vi "MICSD Set Attenuator.vi"(8 "error in (no error)":errorcluster, 10 "Attenuation":u8, 11 "VISA Resource Name":refnum<visa-resource-name>) -> (0 "error out":errorcluster, 3 "dup VISA Resource Name":refnum<visa-resource-name>)   [LabVIEW 2020]
uses:
  <vilib>/Instr/_visa.llb/VISA Configure Serial Port (Instr).vi
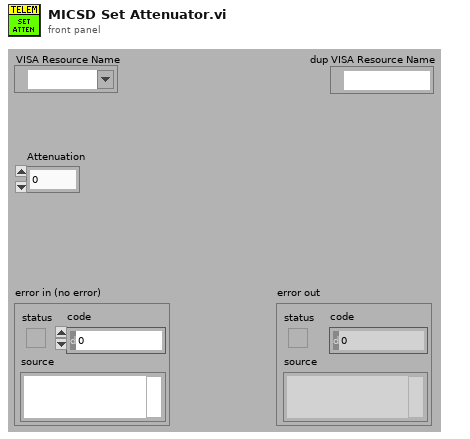
[diagram p1: front panel]
types:
  T1 = cluster{"Command Token":u8, "Length":u16, "Pack Data":u8[]}
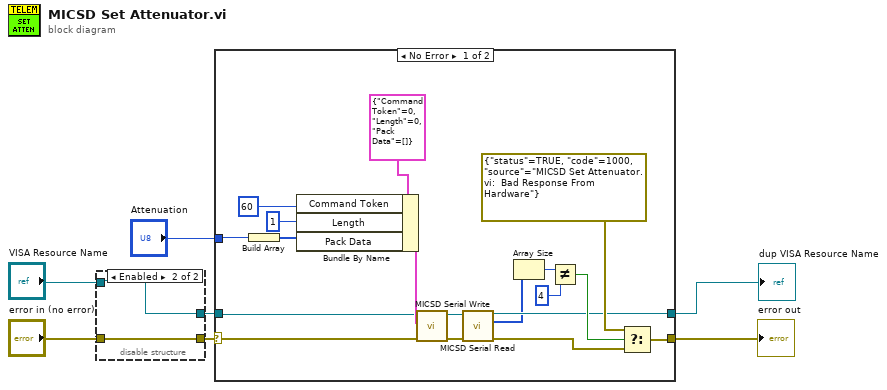
[diagram p0: block diagram]
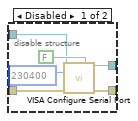
[diagram p2: hidden frame]
diagram:
  n1 = disable-structure shown="Enabled" {
    disable-tunnel: [w11 w14] -> w6
    disable-tunnel: "error in (no error)" -> [w10 w14]
    disable-tunnel: "VISA Resource Name" -> [w9 w15]
    disable-tunnel: [w8 w15] -> w3
    frame Disabled {
      n2 = call-poly "VISA Configure Serial Port"("VISA resource name"=w9, "Enable Termination\nChar (T)"=FALSE ("Enable Termination\nChar (T)"), "baud rate (9600)"=u32 230400, "error in (no error)"=w10) -> ("VISA resource name out"=w8:refnum<visa-resource-name>, "error out"=w11:errorcluster)  [unwired: 10 in]
    }
    frame Enabled {
    }
  }
  n3 = case shown="No Error" w6 {
    selector: w6 -> [w31 w35]
    tunnel: [w18 w35] -> w1
    tunnel: w3 -> [w30 w34]
    tunnel: [w21 w34] -> w7
    tunnel: "Attenuation" -> [w16 _]
    frame No Error {
      n4 = Build Array(w16) -> (w17:u8[])
      n5 = Bundle By Name(cluster=T1 {"Command Token"=0, "Length"=0, "Pack Data"=[]} ("Write Data"), "Command Token"=u16 60 ("Length"), "Length"=u16 1, "Pack Data"=w17) -> (w33:T1)
      n6 = call "MICSD Serial Write.vi"("error in (no error)"=w31, "Write Data"=w33, "VISA Resource Name"=w30) -> ("error out"=w27:errorcluster, "DUP Visa Resource Name"=w28:refnum<visa-resource-name>)  [unwired: 7 in]
      n7 = call "MICSD Serial Read.vi"("error in (no error)"=w27, "VISA Resource Name"=w28) -> ("error out"=w19:errorcluster, "Read Data"=w20:u8[], "DUP Visa Resource Name"=w21:refnum<visa-resource-name>)  [unwired: 7 in]
      n8 = Array Size(array=w20) -> (size(s)=w24:i32)
      n9 = Not Equal?(x=w24, y=4) -> (x != y?=w23:bool)
      n10 = Select(t=errorcluster {"status"=TRUE, "code"=1000, "source"="MICSD Set Attenuator.vi:  Bad Response From Hardware"} ("error IO"), s=w23, f=w19) -> (s? t:f=w18:errorcluster)
    }
    frame Error {
    }
  }
  "dup VISA Resource Name" <- w7
  "error out" <- w1
